vi "Lvi Subsystem Wait Until Done.vi"(8 "error in (no error)":errorcluster, 9 "Timeout":dbl, 11 "TaskRef":i32) -> (0 "error out":errorcluster, 2 "function return":u32(ring), 3 "TaskRef out":i32)   [LabVIEW 2022 SP3, in "DtLvLink.lvlib"]
doc: "Calls directly into the entry points of the DLL of the Data Acq SDK and then waits for the specified task to complete or for the timeout interval (specified by one of the LVI Read or LVI Write VIs) to elapse, whichever comes first. This VI is used by the higher-level VI, DtOLWaitUntilDone."
uses:
  DtLvLink.lvlib
  <userlib>/LV-Link3/DtLvLink_64.dll
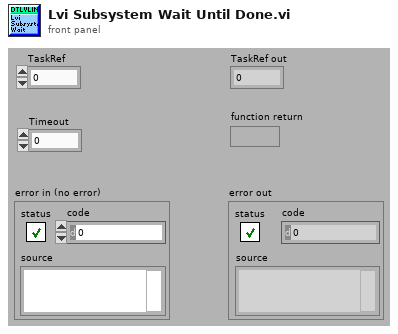
[diagram p1: front panel]
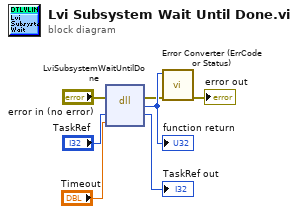
[diagram p0: block diagram]
diagram:
  n1 = dll-call lib="C:/Program Files/National Instruments/LabVIEW 2022/user.lib/LV-Link3/DtLvLink_64.*" fn="LviSubsystemWaitUntilDone"(error in="error in (no error)", "TaskRef"="TaskRef", "Timeout"="Timeout") -> (error out=w3:errorcluster, "return type"=w7:u32, "TaskRef"=→"TaskRef out":i32)  [unwired: 3 in, 1 out]
  "function return" <- w7
  n2 = call "Error Converter (ErrCode or Status).vi"("error in (no error)"=w3, "error code"=w7) -> ("error out"=→"error out":errorcluster)  [unwired: 9 in]
